vi "LIFA io Handler.vi"(0 "Pins":u8[](array[numeric])=[8, 9, 10, 11, 12], 1 "Arduino Resource":T2={"VISA resource"="", "Board Type"=enum."Uno", "Connection Type"=enum."USB / Serial", "Bytes Per Packet (15)"=15}, 2 "Values":u8[](array[numeric]), 4 "error in":errorcluster, 5 "Modes":T1[](array[typedef])=[enum."Output", enum."Output", enum."Output", enum."Output", enum."Output"]) -> (6 "Arduino Resource":T2={"VISA resource"="", "Board Type"=enum."Uno", "Connection Type"=enum."USB / Serial", "Bytes Per Packet (15)"=15}, 8 "error out":errorcluster)   [LabVIEW 2013]
uses:
  <vilib>/LabVIEW Interface for Arduino/Type Defs/Arduino Resource.ctl
  <vilib>/LabVIEW Interface for Arduino/Type Defs/Board Type.ctl
  <vilib>/LabVIEW Interface for Arduino/Type Defs/Pin Mode.ctl
  <vilib>/LabVIEW Interface for Arduino/LabVIEW Interface for Arduino.lvlib
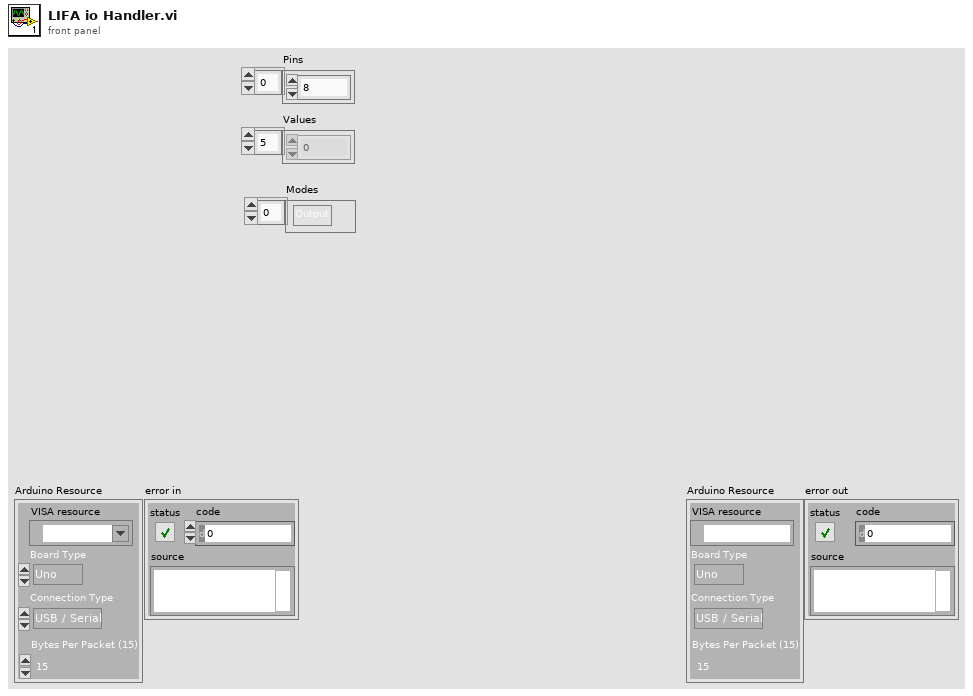
[diagram p1: front panel]
types:
  T1 = typedef "LabVIEW Interface for Arduino.lvlib/Pin Mode.ctl" = enum8{"Input", "Output"}
  T2 = typedef "LabVIEW Interface for Arduino.lvlib/Arduino Resource.ctl" = cluster{"VISA resource":refnum<visa-resource-name>, "Board Type":T3, "Connection Type":enum8{"USB / Serial"}, "Bytes Per Packet (15)":u8}
  T3 = typedef "LabVIEW Interface for Arduino.lvlib/Board Type.ctl" = enum16{"Uno", "Dimuelanove w/Atmega 328", "Mega 2560"}
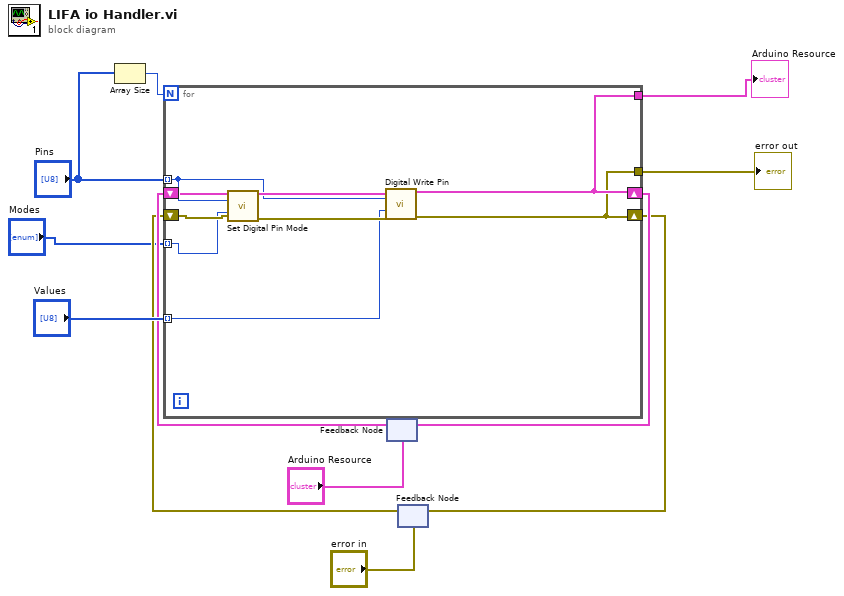
[diagram p0: block diagram]
diagram:
  n1 = Array Size(array="Pins") -> (size(s)=w12:i32)
  n2 = feedback #1("Arduino Resource") -> (w8:T2)
  n3 = feedback #2("error in") -> (w5:errorcluster)
  n4 = for {
    N: w12 -> [_]
    tunnel: "Pins" -> [w19] mode=indexing
    tunnel: "Modes" -> [w13] mode=indexing
    tunnel: "Values" -> [w18] mode=indexing
    shift-right: [w14] -> w6
    shift-left: w5 -> [w16]
    shift-right: [w15] -> w9
    shift-left: w8 -> [w17]
    tunnel: [w15] -> w3
    tunnel: [w14] -> w2
    n5 = call <vilib>:"Set Digital Pin Mode.vi"("Arduino Resource"=w17, "Digital I/O Pin"=w19, "Pin Mode (Input)"=w13, "error in"=w16) -> ("Arduino Resource"=w21:T2, "error out"=w20:errorcluster)  [unwired: 10 in]
    n6 = call <vilib>:"Digital Write Pin.vi"("Arduino Resource"=w21, "Digital I/O Pin (0)"=w19, "Value (0)"=w18, "error in"=w20) -> ("Arduino Resource"=w15:T2, "error out"=w14:errorcluster)  [unwired: 10 in]
  }
  "Arduino Resource" <- w3
  "error out" <- w2
  n7 = feedback-in #1(w9) -> ()
  n8 = feedback-in #2(w6) -> ()
